vi "Tegam4040 - Control [Demo].vi"() -> ()   [LabVIEW 2010]
doc: "Example shows how to use Tegam4040 labVIEW driver"
uses:
  Tegam4040.lvlib
panel:
  in  "Input Impedance":enum16{" 1 MOhm", "50 Ohm"}(ring)
  in  "Calibration":bool
  in  "Attenuation":T1(ring)
  in  "Gain":enum16{"Gain of 1", "Gain of 10", "Gain of 100"}(ring)
  in  "DAC":u16(knob)=32767 scale=0.0..65535.0 scale format="%x"
  in  "Coupling":enum16{"DC Coupling", "AC Coupling"}(ring)
  out "error out":errorcluster
  in  "VISA Tegam4040":refnum<visa-resource-name>
  in  "Low Pass Filter":enum16{"No Filter", "100kHz", "1MHz"}(ring)
  in  "stop":bool
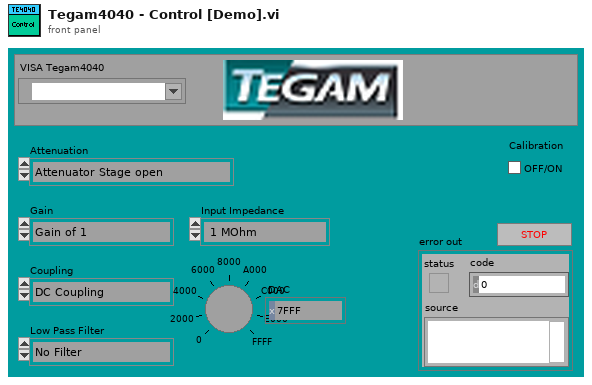
[diagram p1: front panel]
types:
  T1 = enum16{"Attenuator Stage open", "Attenuation of 1", "Attenuation of 10", "Attenuation of 100"}
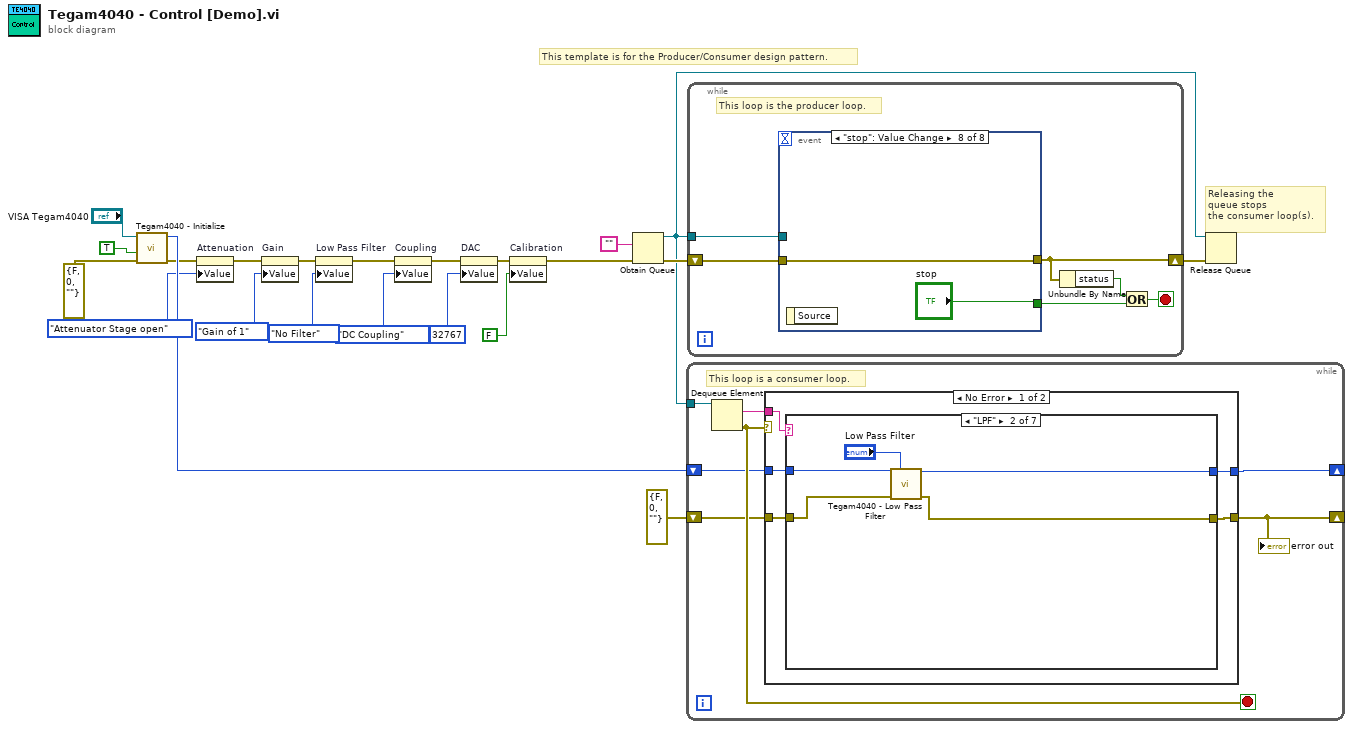
[diagram p0: block diagram]
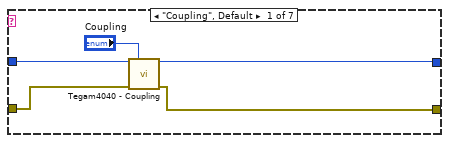
[diagram p2: hidden frame]
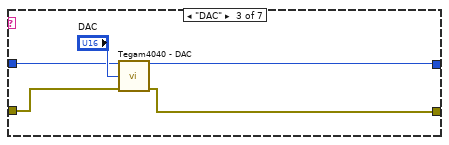
[diagram p3: hidden frame]
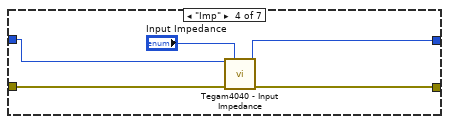
[diagram p4: hidden frame]
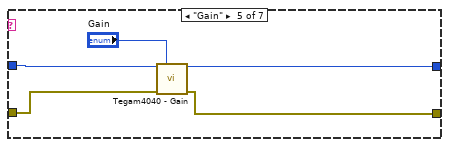
[diagram p5: hidden frame]
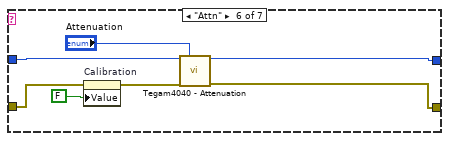
[diagram p6: hidden frame]
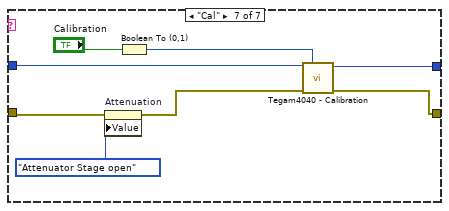
[diagram p7: hidden frame]
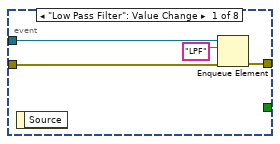
[diagram p9: hidden frame]
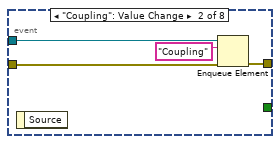
[diagram p10: hidden frame]
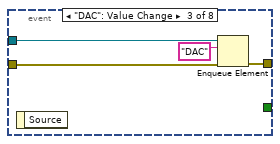
[diagram p11: hidden frame]
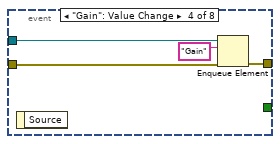
[diagram p12: hidden frame]
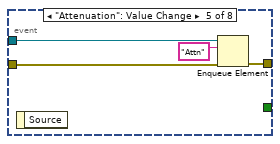
[diagram p13: hidden frame]
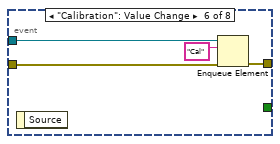
[diagram p14: hidden frame]
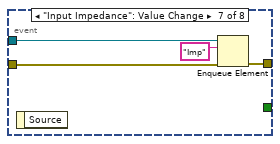
[diagram p15: hidden frame]
diagram:
  # "Releasing the\nqueue stops\nthe consumer loop(s)."
  # "This template is for the Producer/Consumer design pattern."
  n1 = call "Tegam4040 - Initialize.vi"("error in (no error)"=errorcluster {"status"=FALSE, "code"=0, "source"=""}, "Reset? (T: Yes)"=TRUE, "VISA Tegam4040"="VISA Tegam4040") -> ("error out"=w13:errorcluster, "Instrument Session Handle"=w15:u32)  [unwired: 7 in]
  n2 = property on="Attenuation" class="Enum (strict)"(error in=w13, "Value"=T1."Attenuator Stage open" ("Attenuation")) -> (error out=w3:errorcluster)  [unwired: 1 in, 1 out]
  n3 = property on="Gain" class="Enum (strict)"(error in=w3, "Value"=enum16{"Gain of 1", "Gain of 10", "Gain of 100"}."Gain of 1" ("Gain")) -> (error out=w2:errorcluster)  [unwired: 1 in, 1 out]
  n4 = property on="Low Pass Filter" class="Enum (strict)"(error in=w2, "Value"=enum16{"No Filter", "100kHz", "1MHz"}."No Filter" ("Low Pass Filter")) -> (error out=w1:errorcluster)  [unwired: 1 in, 1 out]
  n5 = property on="Coupling" class="Enum (strict)"(error in=w1, "Value"=enum16{"DC Coupling", "AC Coupling"}."DC Coupling" ("Coupling")) -> (error out=w8:errorcluster)  [unwired: 1 in, 1 out]
  n6 = property on="DAC" class="Knob (strict)"(error in=w8, "Value"=u32 32767 ("DAC")) -> (error out=w6:errorcluster)  [unwired: 1 in, 1 out]
  n7 = property on="Calibration" class="Bool (strict)"(error in=w6, "Value"=FALSE ("Calibration")) -> (error out=w4:errorcluster)  [unwired: 1 in, 1 out]
  n8 = Obtain Queue(element data type="" ("data (can be any type)"), error in (no error)=w4) -> (queue out=w19:refnum<queue>, error out=w22:errorcluster)  [unwired: 3 in, 1 out]
  n9 = while {
    tunnel: w19 -> [w29]
    shift-right: [w25] -> _
    shift-left: w15 -> [w26]
    shift-right: [w23] -> _
    shift-left: errorcluster {"status"=FALSE, "code"=0, "source"=""} ("error out") -> [w24]
    stop <- w28 stop-if-true
    # "This loop is a consumer loop."
    n10 = Dequeue Element(queue=w29) -> (element=w27:string, error out=w28:errorcluster)  [unwired: 2 in, 2 out]
    n11 = case shown="No Error" w28 {
      tunnel: w27 -> [w34 _]
      tunnel: w26 -> [w33 w75]
      tunnel: [w32 w75] -> w25
      tunnel: w24 -> [w31 w76]
      tunnel: [w30 w76] -> w23
      frame No Error {
        n12 = case shown="\"LPF\"" w34 {
          tunnel: w33 -> [w38 w44 w48 w53 w58 w65 w74]
          tunnel: [w37 w43 w47 w50 w57 w64 w69] -> w32
          tunnel: w31 -> [w36 w41 w45 w52 w56 w63 w72]
          tunnel: [w35 w40 w46 w51 w55 w60 w70] -> w30
          frame "Coupling", Default {
            n13 = call "Tegam4040 - Coupling.vi"("Instrument Session Handle In"=w38, "Coupling"="Coupling", "error in (no error)"=w36) -> ("Instrument Session Handle Out (dupl)"=w37:u32, "error out"=w35:errorcluster)  [unwired: 11 in]
          }
          frame "LPF" {
            n14 = call "Tegam4040 - Low Pass Filter.vi"("Instrument Session Handle In"=w44, "LP Filter"="Low Pass Filter", "error in (no error)"=w41) -> ("Instrument Session Handle Out (dupl)"=w43:u32, "error out"=w40:errorcluster)  [unwired: 11 in]
          }
          frame "DAC" {
            n15 = call "Tegam4040 - DAC.vi"("Instrument Session Handle In"=w48, "DAC"="DAC", "error in (no error)"=w45) -> ("Instrument Session Handle Out (dupl)"=w47:u32, "error out"=w46:errorcluster)  [unwired: 11 in]
          }
          frame "Imp" {
            n16 = call "Tegam4040 - Input Impedance.vi"("Instrument Session Handle In"=w53, "Input Impedance"="Input Impedance", "error in (no error)"=w52) -> ("Instrument Session Handle Out (dupl)"=w50:u32, "error out"=w51:errorcluster)  [unwired: 11 in]
          }
          frame "Gain" {
            n17 = call "Tegam4040 - Gain.vi"("Instrument Session Handle In"=w58, "Gain"="Gain", "error in (no error)"=w56) -> ("Instrument Session Handle Out (dupl)"=w57:u32, "error out"=w55:errorcluster)  [unwired: 11 in]
          }
          frame "Attn" {
            n18 = property on="Calibration" class="Bool (strict)"(error in=w63, "Value"=FALSE ("Calibration")) -> (error out=w62:errorcluster)  [unwired: 1 in, 1 out]
            n19 = call "Tegam4040 - Attenuation.vi"("Instrument Session Handle In"=w65, "Attenuation"="Attenuation", "error in (no error)"=w62) -> ("Instrument Session Handle Out (dupl)"=w64:u32, "error out"=w60:errorcluster)  [unwired: 11 in]
          }
          frame "Cal" {
            n20 = property on="Attenuation" class="Enum (strict)"(error in=w72, "Value"=T1."Attenuator Stage open" ("Attenuation")) -> (error out=w71:errorcluster)  [unwired: 1 in, 1 out]
            n21 = Boolean To (0,1)(Boolean="Calibration") -> (0, 1=w67:i16)
            n22 = call "Tegam4040 - Calibration.vi"("Instrument Session Handle In"=w74, "Calibration"=w67, "error in (no error)"=w71) -> ("Instrument Session Handle Out (dupl)"=w69:u32, "error out"=w70:errorcluster)  [unwired: 11 in]
          }
        }
      }
      frame Error {
      }
    }
    "error out" <- w23
  }
  n23 = while {
    shift-right: [w78] -> w21
    shift-left: w22 -> [w81]
    tunnel: w19 -> [w82]
    stop <- w79 stop-if-true
    # "This loop is the producer loop."
    n24 = event shown="[7] \"stop\": Value Change" {
      selector: _ -> [_ _ _ _ _ _ _ _]
      dyn-events: _ -> [_ _ _ _ _ _ _ _]
      timeout: _ -> [_ _ _ _ _ _ _ _]
      tunnel: w82 -> [w86 w90 w94 w98 w102 w106 w110 _]
      tunnel: w81 -> [w85 w89 w93 w97 w101 w105 w109 w111]
      tunnel: [w84 w88 w92 w96 w100 w104 w108 w111] -> w78
      tunnel: [_ _ _ _ _ _ _ "stop"] -> w80
      event "Low Pass Filter": Value Change {
        n25 = event-data() -> ()  [unwired: 1 in, 1 out]
        n26 = Enqueue Element(queue=w86, element="LPF", error in (no error)=w85) -> (error out=w84:errorcluster)  [unwired: 1 in, 2 out]
      }
      event "Coupling": Value Change {
        n27 = event-data() -> ()  [unwired: 1 in, 1 out]
        n28 = Enqueue Element(queue=w90, element="Coupling", error in (no error)=w89) -> (error out=w88:errorcluster)  [unwired: 1 in, 2 out]
      }
      event "DAC": Value Change {
        n29 = event-data() -> ()  [unwired: 1 in, 1 out]
        n30 = Enqueue Element(queue=w94, element="DAC", error in (no error)=w93) -> (error out=w92:errorcluster)  [unwired: 1 in, 2 out]
      }
      event "Gain": Value Change {
        n31 = event-data() -> ()  [unwired: 1 in, 1 out]
        n32 = Enqueue Element(queue=w98, element="Gain", error in (no error)=w97) -> (error out=w96:errorcluster)  [unwired: 1 in, 2 out]
      }
      event "Attenuation": Value Change {
        n33 = event-data() -> ()  [unwired: 1 in, 1 out]
        n34 = Enqueue Element(queue=w102, element="Attn", error in (no error)=w101) -> (error out=w100:errorcluster)  [unwired: 1 in, 2 out]
      }
      event "Calibration": Value Change {
        n35 = event-data() -> ()  [unwired: 1 in, 1 out]
        n36 = Enqueue Element(queue=w106, element="Cal", error in (no error)=w105) -> (error out=w104:errorcluster)  [unwired: 1 in, 2 out]
      }
      event "Input Impedance": Value Change {
        n37 = event-data() -> ()  [unwired: 1 in, 1 out]
        n38 = Enqueue Element(queue=w110, element="Imp", error in (no error)=w109) -> (error out=w108:errorcluster)  [unwired: 1 in, 2 out]
      }
      event "stop": Value Change {
        n39 = event-data() -> ()  [unwired: 1 in, 1 out]
      }
    }
    n40 = Unbundle By Name(w78) -> ("status"=w77:bool)
    n41 = Or(x=w77, y=w80) -> (x .or. y?=w79:bool)
  }
  n42 = Release Queue(queue=w19, error in (no error)=w21) -> ()  [unwired: 1 in, 3 out]
